vi "correccioncentroide.vi"(0 "Toma Original":T1, 1 "Patrón original":T1) -> (2 "Tom trasladada":T1(plugin-control) caption="Perfil lateral", 3 "Patron original(dup)":T1(plugin-control), 4 "Centroide Captura":cluster{"X Centroid":sgl, "Y Centroid":sgl}, 5 "Centroide Patron":cluster{"X Centroid":sgl, "Y Centroid":sgl})   [LabVIEW 2021]
doc: "Traslada una imagen con respecto a otra haciendo coincidir sus centroides"
uses:
  <vilib>/vision/Image Controls.llb/IMAQ Image.ctl
  <vilib>/vision/NI_Vision_Development_Module.lvlib
panel:
  # "CUEVAS CERÓN SERGIO ALBERTO\nREYES PÉREZ JAVIER\nSALCEDO LICEA JUAN CARLOS"
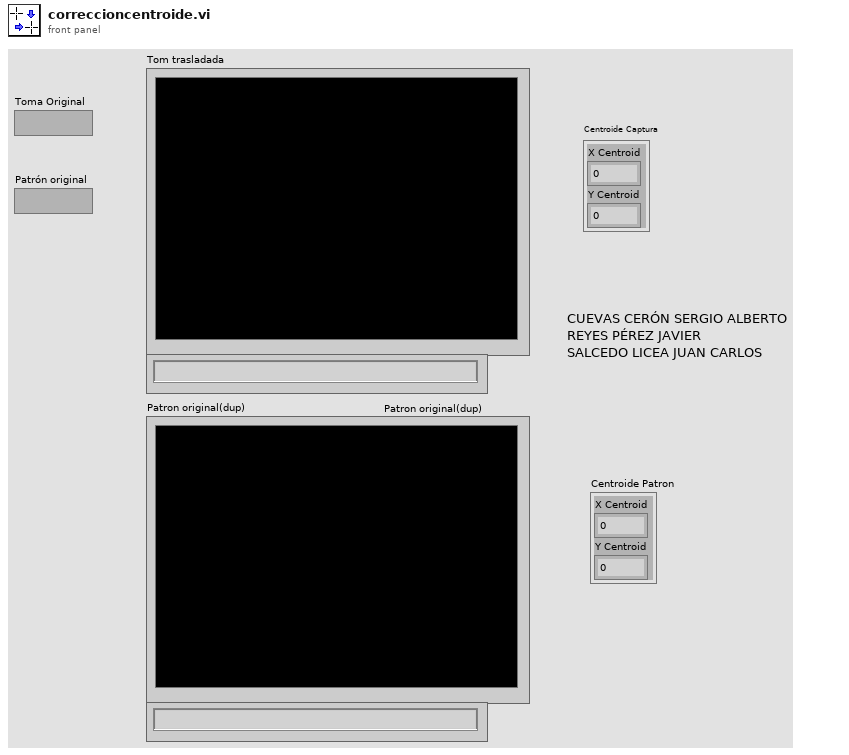
[diagram p1: front panel]
types:
  T1 = typedef "IMAQ Image.ctl" = refnum<image>
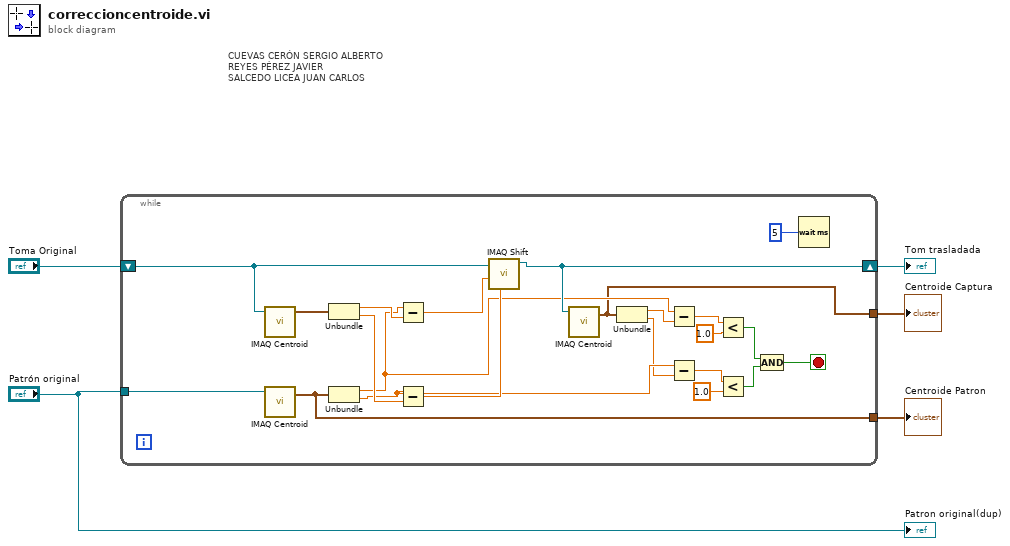
[diagram p0: block diagram]
diagram:
  # "CUEVAS CERÓN SERGIO ALBERTO\nREYES PÉREZ JAVIER\nSALCEDO LICEA JUAN CARLOS"
  n1 = while {
    tunnel: "Patrón original" -> [w14]
    shift-right: [w25] -> w5
    shift-left: "Toma Original" -> [w15]
    tunnel: [w7] -> w2
    tunnel: [w6] -> w1
    stop <- w16 stop-if-true
    n2 = call "IMAQ Centroid"("Image"=w15) -> ("Centroid"=w8:cluster{"X Centroid":sgl, "Y Centroid":sgl})  [unwired: 3 in, 1 out]
    n3 = call "IMAQ Centroid"("Image"=w14) -> ("Centroid"=w6:cluster{"X Centroid":sgl, "Y Centroid":sgl})  [unwired: 3 in, 1 out]
    n4 = Unbundle(w8) -> ("X Centroid"=w24:sgl, "Y Centroid"=w23:sgl)
    n5 = Unbundle(w6) -> ("X Centroid"=w21:sgl, "Y Centroid"=w22:sgl)
    n6 = Subtract(x=w21, y=w24) -> (x-y=w26:sgl)
    n7 = Subtract(x=w22, y=w23) -> (x-y=w27:sgl)
    n8 = call "IMAQ Shift"("YOffset"=w27, "XOffset"=w26, "Image Src"=w15) -> ("Image Dst Out"=w25:T1)  [unwired: 7 in, 1 out]
    n9 = call "IMAQ Centroid"("Image"=w25) -> ("Centroid"=w7:cluster{"X Centroid":sgl, "Y Centroid":sgl})  [unwired: 3 in, 1 out]
    n10 = Unbundle(w7) -> ("X Centroid"=w11:sgl, "Y Centroid"=w10:sgl)
    n11 = Subtract(x=w21, y=w11) -> (x-y=w13:sgl)
    n12 = Subtract(x=w22, y=w10) -> (x-y=w12:sgl)
    n13 = Less?(x=w13, y=sgl 1.0) -> (x < y?=w17:bool)
    n14 = Less?(x=w12, y=sgl 1.0) -> (x < y?=w18:bool)
    n15 = Compound Arithmetic op=AND(w17, w18) -> (w16:bool)
    n16 = Wait (ms)(milliseconds to wait=u32 5) -> ()  [unwired: 1 out]
  }
  "Tom trasladada" <- w5
  "Centroide Captura" <- w2
  "Centroide Patron" <- w1
  "Patron original(dup)" <- "Patrón original"
